vi "RWNoise-Compute.vi"(0 "RW Noise Params":T1, 7 "Spectrum (uV)":dbl[](array[numeric]), 11 "error in (no error)":errorcluster) -> (6 "RW Noise (uV)":dbl, 10 "Spectrum (uV/sqrt(Hz))":waveform(dbl), 15 "error out":errorcluster)   [LabVIEW 2020]
uses:
  RWNoise Params.ctl
  epl-vi-lib/Utility VIs/Type Defs/Left-Right ring.ctl
  <vilib>/Analysis/NI_AALPro.lvlib
  <vilib>/Analysis/5stat.llb/RMS (DBL).vi
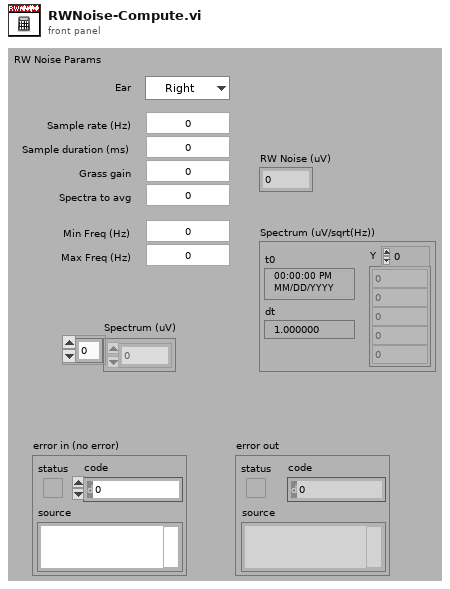
[diagram p1: front panel]
types:
  T1 = typedef "RWNoise Params.ctl" = cluster{"Sample rate (Hz)":dbl, "Sample duration (ms)":dbl, "Grass gain":dbl, "Min Freq (Hz)":dbl, "Max Freq (Hz)":dbl, "Spectra to avg":i32, "Ear":T2}
  T2 = typedef "Left-Right ring.ctl" = enum16{"Right", "Left"}
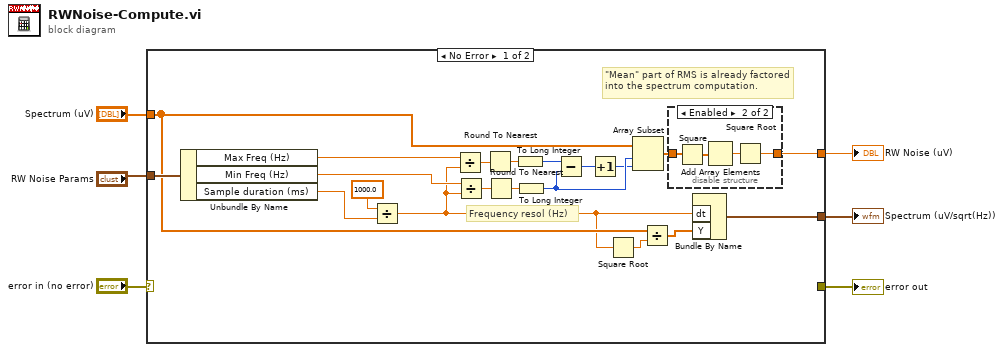
[diagram p0: block diagram]
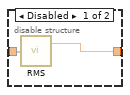
[diagram p2: hidden frame]
diagram:
  n1 = case shown="No Error" "error in (no error)" {
    selector: "error in (no error)" -> [_ w33]
    tunnel: "RW Noise Params" -> [w26 _]
    tunnel: "Spectrum (uV)" -> [w11 _]
    tunnel: [w12 _] -> w3
    tunnel: [w10 _] -> w2
    tunnel: [_ w33] -> w1
    frame No Error {
      # "\"Mean\" part of RMS is already factored into the spectrum computation."
      # "Frequency resol (Hz)"
      n2 = Unbundle By Name(w26) -> ("Max Freq (Hz)"=w23:dbl, "Min Freq (Hz)"=w22:dbl, "Sample duration (ms)"=w25:dbl)
      n3 = Divide(x=1000.0, y=w25) -> (x/y=w7:dbl)
      n4 = Divide(x=w23, y=w7) -> (x/y=w21:dbl)
      n5 = Divide(x=w22, y=w7) -> (x/y=w20:dbl)
      n6 = Round To Nearest(number=w21) -> (nearest integer value=w19:dbl)
      n7 = Round To Nearest(number=w20) -> (nearest integer value=w18:dbl)
      n8 = To Long Integer(number=w19) -> (32bit integer=w17:i32)
      n9 = To Long Integer(number=w18) -> (32bit integer=w15:i32)
      n10 = Subtract(x=w17, y=w15) -> (x-y=w16:i32)
      n11 = Increment(x=w16) -> (x+1=w14:i32)
      n12 = Square Root(x=w7) -> (sqrt(x)=w8:dbl)
      n13 = Array Subset(array=w11, index=w15, length=w14) -> (w13:dbl[])
      n14 = Divide(x=w11, y=w8) -> (x/y=w9:dbl[])
      n15 = disable-structure shown="Enabled" {
        disable-tunnel: w13 -> [w28 w32]
        disable-tunnel: [w27 w29] -> w12
        frame Disabled {
          n16 = call-poly <vilib>:"RMS.vi"("X"=w28) -> ("rms value"=w27:dbl)  [unwired: 1 out]
        }
        frame Enabled {
          n17 = Square(x=w32) -> (x^2=w31:dbl[])
          n18 = Add Array Elements(numeric array=w31) -> (sum=w30:dbl)
          n19 = Square Root(x=w30) -> (sqrt(x)=w29:dbl)
        }
      }
      n20 = Bundle By Name("dt"=w7, "Y"=w9) -> (w10:waveform(dbl))  [unwired: 1 in]
    }
    frame Error {
    }
  }
  "error out" <- w1
  "RW Noise (uV)" <- w3
  "Spectrum (uV/sqrt(Hz))" <- w2
